vi "Create All Message Queues.vi"(8 "error in (no error)":errorcluster) -> (0 "error out":errorcluster, 3 "Message Queues out":T1)   [LabVIEW 2015, in "Message Queue.lvlib"]
doc: "This VI creates and initializes all the message queues for your application. If your application requires more than one message queue, right-click the \"Message Queues\" constant above and select Open Type Def. Add the new Message Queue(s) to the type definition, then initialize them in this VI."
uses:
  Message Queue.lvlib
  All Message Queues.ctl
  Message Cluster.ctl
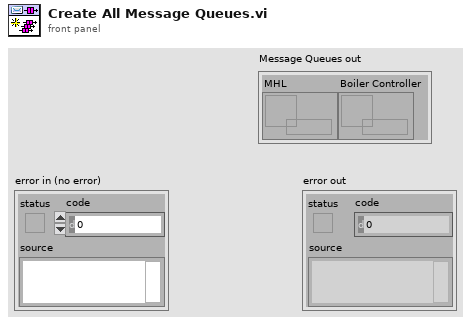
[diagram p1: front panel]
types:
  T1 = typedef "Message Queue.lvlib/All Message Queues.ctl" = cluster{"MHL":refnum<queue>, "Boiler Controller":refnum<queue>}
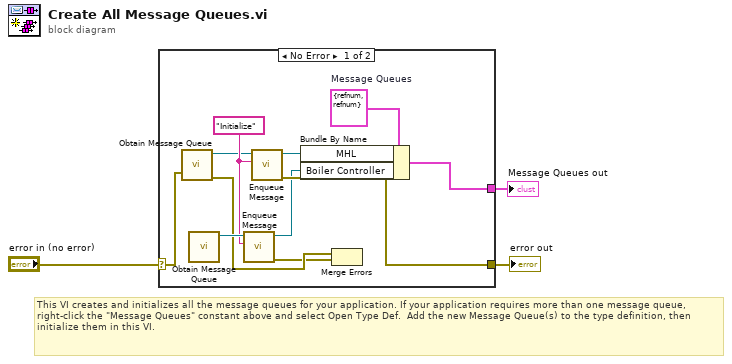
[diagram p0: block diagram]
diagram:
  # "This VI creates and initializes all the message queues for your application. If your application requires more than one message queue, right-click the \"Message Queues\" constant above and select Open Type Def.  Add the new Message Queue(s) to the type definition, then initialize them in this VI."
  n1 = case shown="No Error" "error in (no error)" {
    selector: "error in (no error)" -> [w12 w15]
    tunnel: [w14 w15] -> w3
    tunnel: [w13 _] -> w2
    frame No Error {
      w10 = "Initialize" ("Message")
      w5 = T1 {"MHL"=refnum, "Boiler Controller"=refnum}  # Message Queues
      n2 = call "Obtain Message Queue.vi"("error in (no error)"=w12) -> ("error out"=w6:errorcluster, "Message Queue"=w8:refnum<queue>)  [unwired: 9 in]
      n3 = call "Obtain Message Queue.vi"() -> ("Message Queue"=w11:refnum<queue>)  [unwired: 10 in, 1 out]
      n4 = call "Enqueue Message.vi"("Message"=w10, "Message Queue"=w11) -> ("error out"=w4:errorcluster, "dup Message Queue"=w7:refnum<queue>)  [unwired: 8 in]
      n5 = call "Enqueue Message.vi"("Message"=w10, "Message Queue"=w8) -> ("error out"=w14:errorcluster, "dup Message Queue"=w9:refnum<queue>)  [unwired: 8 in]
      n6 = Bundle By Name(cluster=w5, "MHL"=w9, "Boiler Controller"=w7) -> (w13:T1)
      n7 = Merge Errors(w6, w4) -> ()  [unwired: 1 out]
    }
    frame Error {
    }
  }
  "Message Queues out" <- w2
  "error out" <- w3
